vi "Image Compression with PCA.vi"() -> ()   [LabVIEW 2023]
doc: "This example shows the application of principal component analysis (PCA) in image compression.\n\nYou can consider each row of the image as a time series and the whole image as a multivariate time series. After applying PCA, the correlation among the rows of the image is reduced. Only a few rows of the resulting principal component scores contain significant information. By keeping only the rows with important information, you can reduce the dimensionality of the image and retain important information of the image. \n\nThis example uses the TSA Principal Component Analysis VI to compute principal component scores of an image and reconstruct the image with only part of the principal component scores that contain significant or useful values.\n\n<b>Instructions:</b>\n1) Run this VI.\n2) Change the number of rows to keep principal component scores with significant information and observe the PSNR of the image."
uses:
  <vilib>/Analysis/baseanly.llb/Real A x B.vi
  <vilib>/addons/Time Series Analysis/Statistical Analysis.llb/TSA Principal Component Analysis (Array).vi
  <vilib>/Analysis/Matrix/Numeric/Conversions/Matrix To Array - RM.vi
  <vilib>/addons/_Advanced Signal Processing/NI_AdvSigProcTSA.lvlib
  <vilib>/Analysis/NI_AALBase.lvlib
  <vilib>/Analysis/Matrix/NI_Matrix.lvlib
panel:
  in  "Number of rows to keep":i32=50
  out "PSNR (dB)":dbl=35.02134881593631
  out "X-Ray Image":dbl[][](graph)
  out "Principal Component Scores":dbl[][](graph)
  out "Reconstructed Image":dbl[][](graph)
  in  "stop":bool
  # "Overview: Shows the application of principal component analysis (PCA) in image compression.\nRequirements: LabVIEW Full Development System, Advanced Signal Processing Toolkit\nInstructions: \n1. Run this VI.\n2. Change the number of rows to keep principal component scores with significant information and observe the PSNR of the image.\n3. Click Stop to stop the VI."
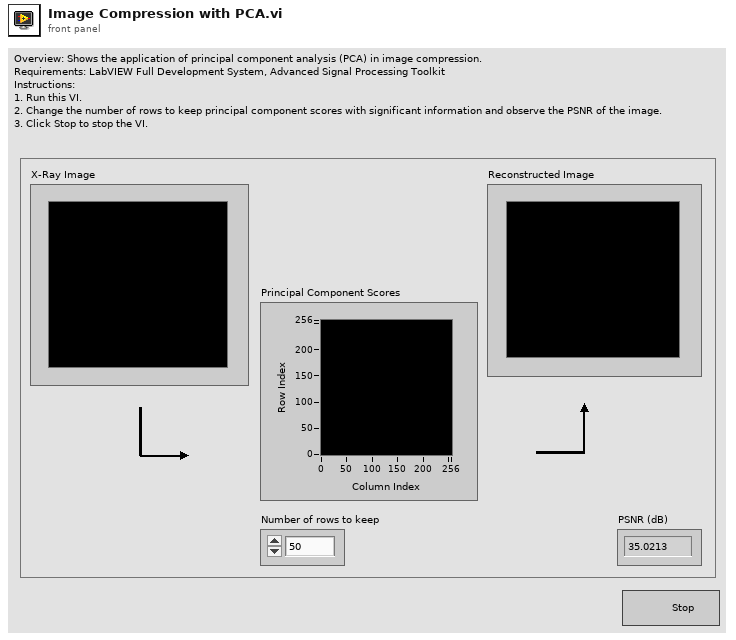
[diagram p1: front panel]
types:
  T1 = typedef "NI_Matrix.lvlib/RealMatrix.ctl" = dbl[][]
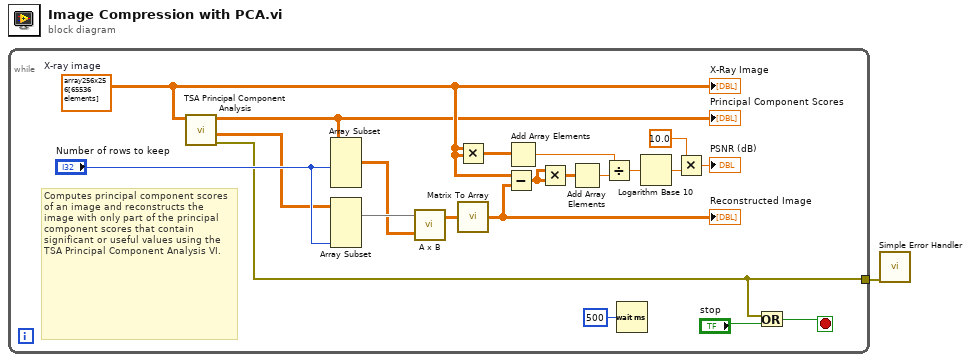
[diagram p0: block diagram]
diagram:
  n1 = while {
    tunnel: [w2] -> w1
    stop <- w16 stop-if-true
    w6 = dbl[][] array256x256[65536 elements]  # X-ray image
    # "Computes principal component scores of an image and reconstructs the image with only part of the principal component scores that contain significant or useful values using the TSA Principal Component Analysis VI."
    n2 = call-poly <vilib>:"TSA Principal Component Analysis.vi"("Xt"=w6) -> ("error out"=w2:errorcluster, "weights"=w19:dbl[][], "Xt out"=w5:dbl[][])  [unwired: 2 in, 6 out]
    "Principal Component Scores" <- w5
    n3 = Array Subset(array=w5, length (row)="Number of rows to keep") -> (w17:dbl[][])  [unwired: 3 in]
    n4 = Array Subset(array=w19, length (col)="Number of rows to keep") -> (w18:dbl[][])  [unwired: 3 in]
    n5 = call-poly <vilib>:"A x B.vi"("B"=w17, "A"=w18) -> ("A x B"=w4:T1)  [unwired: 1 out]
    n6 = Multiply(x=w6, y=w6) -> (x*y=w12:dbl[][])
    n7 = call-poly <vilib>:"Matrix To Array.vi"("Real Matrix"=w4) -> ("Real 2D Array"=w3:dbl[][])
    "Reconstructed Image" <- w3
    n8 = Subtract(x=w6, y=w3) -> (x-y=w13:dbl[][])
    n9 = Add Array Elements(numeric array=w12) -> (sum=w7:dbl)
    n10 = Multiply(x=w13, y=w13) -> (x*y=w14:dbl[][])
    n11 = Add Array Elements(numeric array=w14) -> (sum=w11:dbl)
    n12 = Divide(x=w7, y=w11) -> (x/y=w10:dbl)
    n13 = Wait (ms)(milliseconds to wait=u32 500 ("millisecond multiple")) -> ()  [unwired: 1 out]
    n14 = Logarithm Base 10(1:w10) -> (0:w9:dbl)
    n15 = Multiply(x=10.0, y=w9) -> (x*y=→"PSNR (dB)":dbl)
    n16 = Or(x=w2, y="stop") -> (x .or. y?=w16:bool)
    "X-Ray Image" <- w6
  }
  n17 = call <vilib>:"Simple Error Handler.vi"("error in (no error)"=w1) -> ()  [unwired: 1 in, 8 out]
